vi "Get Refnum.vi"(8 "error in (no error)":errorcluster, 11 "Ctrl Refnum Value Source in":refnum<class "Ctrl Refnum Value Source.lvclass">) -> (0 "error out":errorcluster, 2 "Refnum":variant, 3 "Ctrl Refnum Value Source out":refnum<class "Ctrl Refnum Value Source.lvclass">)   [LabVIEW 2020, in "Composed Columns.lvlib" / "Ctrl Refnum Value Source.lvclass"]
uses:
  Ctrl Refnum Value Source.lvclass
  Ctrl Refnum Value Source.lvclass/Ctrl Refnum Value Source.ctl
panel:
  # "Here I use a variant because\nDVR and refnum are both type\nspecific"
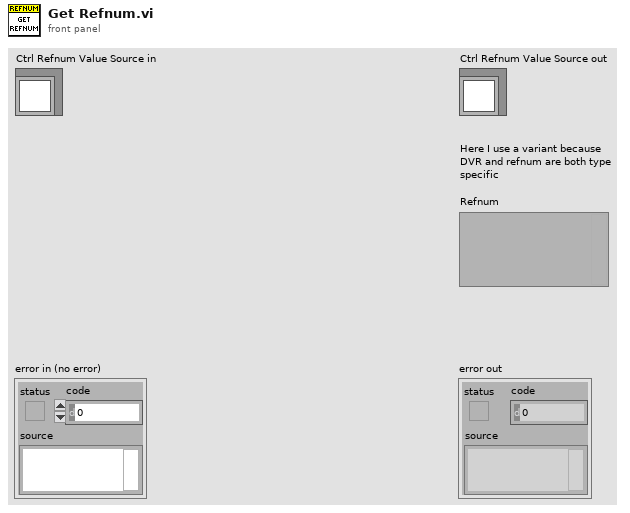
[diagram p1: front panel]
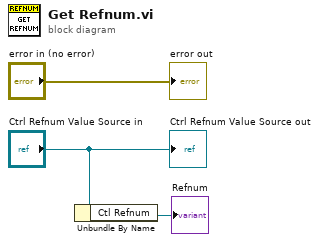
[diagram p0: block diagram]
diagram:
  n1 = Unbundle By Name("Ctrl Refnum Value Source in") -> ("Ctl Refnum"=→"Refnum":refnum<vi>)
  "error out" <- "error in (no error)"
  "Ctrl Refnum Value Source out" <- "Ctrl Refnum Value Source in"
